vi "Unflatten JSONpath Array to Object.vi"(8 "error in (no error)":errorcluster, 9 "JSON Items":string[](array[string]), 10 "Initial JSON Object":string="{}", 11 "$Paths":string[](array[string])) -> (0 "error out":errorcluster, 3 "<JSON>":string)   [LabVIEW 2021, in "jsontext.facade.lvlib"]
doc: "Takes arrays of $Paths items and generates a Object containing those $Paths. Does not support multi-point paths.\n\nFor example: the $Paths (Items):\n$.A.B1 (1)\n$.A.B2 (\"x\")\n$.A2 (true)\n$.A3.C (123)\nproduce the JSON: {\"A\":{\"B1\":1\"B2:\"x\"},\"A2\":true,\"A3\":{\"C\":123}}"
uses:
  jsontext.facade.lvlib
  jsontext/JSONtext.lvlib
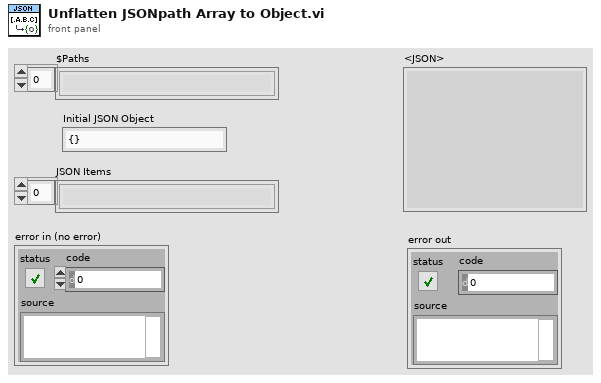
[diagram p1: front panel]
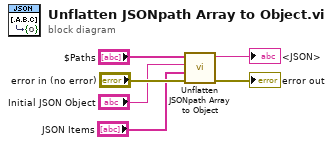
[diagram p0: block diagram]
diagram:
  n1 = call "Unflatten JSONpath Array to Object.vi"("error in (no error)"="error in (no error)", "JSON Items"="JSON Items", "Initial JSON Object"="Initial JSON Object", "$Paths"="$Paths") -> ("error out"=→"error out":errorcluster, "<JSON>"=→"<JSON>":string)  [unwired: 6 in]
